vi "VIE.Module.Queued Message Handler.QueuedMessageHandler_setModifiedData(RemoveLocked).vi"(0 "reference":T1, 2 "data":T2, 5 "error in (no error)":errorcluster) -> (14 "duplicate reference":T1, 19 "error out":errorcluster)   [LabVIEW 2010, in "VIE.Module.Queued Message Handler.QueuedMessageHandler.dqGOOPClass.lvlib"]
doc: "This VI writes the data of the dqGOOP object and unlocks it for write access. In addition, the locked data is removed from the cache."
uses:
  VIE.Module.Queued Message Handler.QueuedMessageHandler.dqGOOPClass.lvlib
  VIE.Module.Queued Message Handler.dqClass_ObjectReference.ctl
  VIE.Module.Queued Message Handler.dqClass_ObjectData.ctl
panel:
  in  "queue (default)":refnum<queue>
  # "Copyright (C) 2004 DataAct Incorporated"
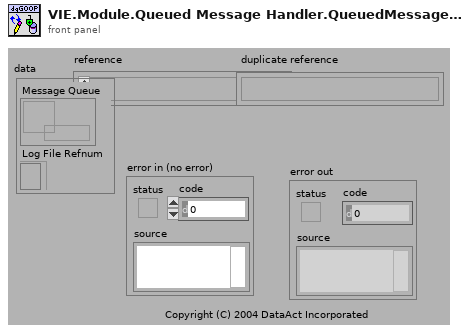
[diagram p1: front panel]
types:
  T1 = typedef "VIE.Module.Queued Message Handler.QueuedMessageHandler.dqGOOPClass.lvlib/VIE.Module.Queued Message Handler.dqClass_ObjectReference.ctl" = refnum<k1>
  T2 = typedef "VIE.Module.Queued Message Handler.QueuedMessageHandler.dqGOOPClass.lvlib/VIE.Module.Queued Message Handler.dqClass_ObjectData.ctl" = cluster{"Message Queue":refnum<queue>, "Log File Refnum":refnum<file>}
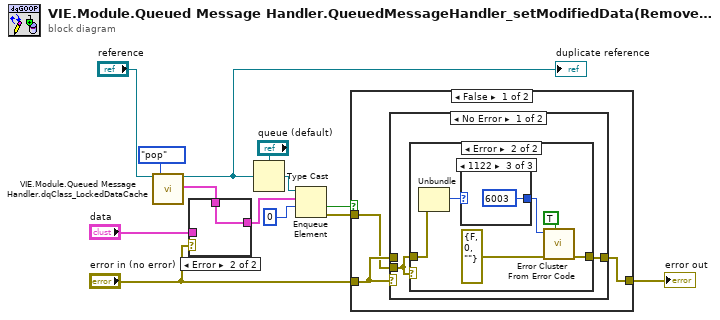
[diagram p0: block diagram]
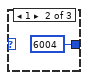
[diagram p5: hidden frame]
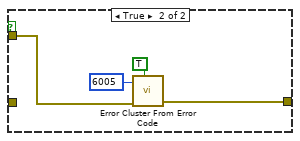
[diagram p7: hidden frame]
diagram:
  n1 = call "VIE.Module.Queued Message Handler.dqClass_LockedDataCache.vi"("reference"="reference", "action (read)"=enum16{"push", "read", "pop"}."pop" ("action")) -> ("reference dup"=w2:T1, "data out"=w4:T2)  [unwired: 14 in, 2 out]
  "duplicate reference" <- w2
  n2 = case shown="Error" "error in (no error)" {
    tunnel: [w14 w15] -> w10
    tunnel: "data" -> [w14 _]
    tunnel: w4 -> [_ w15]
    frame No Error {
    }
    frame Error {
    }
  }
  n3 = Type Cast(type="queue (default)", x=w2) -> (*(type *) &x=w7:refnum<queue>)
  n4 = Enqueue Element(queue=w7, element=w10, timeout in ms (-1)=0 ("timeout in ms (0)")) -> (timed out?=w12:bool, error out=w6:errorcluster)  [unwired: 1 in, 1 out]
  n5 = case shown="False" w12 {
    tunnel: "error in (no error)" -> [w18 _]
    tunnel: [w17 w34] -> w13
    tunnel: w6 -> [w16 w32]
    frame False {
      n6 = case shown="No Error" w18 {
        tunnel: [w19 w31] -> w17
        tunnel: w18 -> [_ w31]
        tunnel: w16 -> [w20 _]
        frame No Error {
          n7 = case shown="Error" w20 {
            tunnel: [w21 w22] -> w19
            tunnel: w20 -> [w21 w27]
            frame No Error {
            }
            frame Error {
              n8 = Unbundle(w27) -> ("code"=w26:i32)  [unwired: 2 out]
              n9 = case shown="1122" w26 {
                selector: w26 -> [w28 _ _]
                tunnel: [w28 6004 ("code") 6003 ("code")] -> w24
                frame Default {
                }
                frame 1 {
                }
                frame 1122 {
                }
              }
              n10 = call <vilib>:"Error Cluster From Error Code.vi"("show call chain? (False)"=TRUE, "error in (no error)"=errorcluster {"status"=FALSE, "code"=0, "source"=""} ("error out"), "error code (0)"=w24) -> ("error out"=w22:errorcluster)  [unwired: 6 in]
            }
          }
        }
        frame Error {
        }
      }
    }
    frame True {
      n11 = call <vilib>:"Error Cluster From Error Code.vi"("show call chain? (False)"=TRUE, "error in (no error)"=w32, "error code (0)"=6005 ("code")) -> ("error out"=w34:errorcluster)  [unwired: 6 in]
    }
  }
  "error out" <- w13
